vi "CalcHum.vi"(8 "error in (no error)":errorcluster, 10 "Adc_Hum":i32, 11 "BME68x in":refnum<class "BME680.lvclass">) -> (0 "error out":errorcluster, 2 "Hum":i32, 3 "BME68x out":refnum<class "BME680.lvclass">)   [LabVIEW 2022 SP3, in "BME680.lvlib" / "BME680.lvclass"]
uses:
  BME680.lvclass
  BME680.lvclass/BME680.ctl
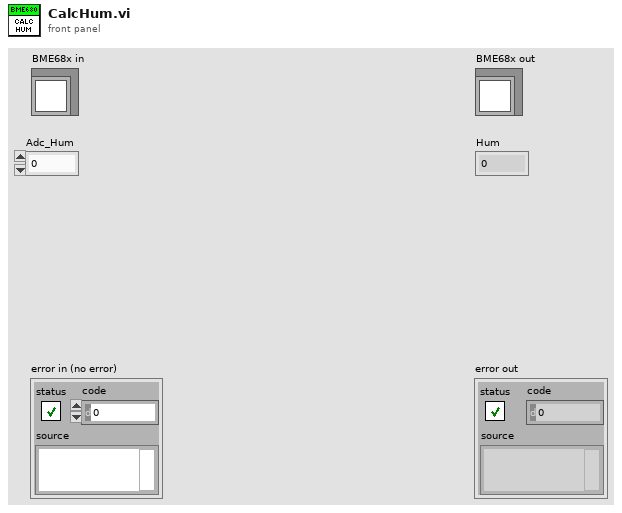
[diagram p1: front panel]
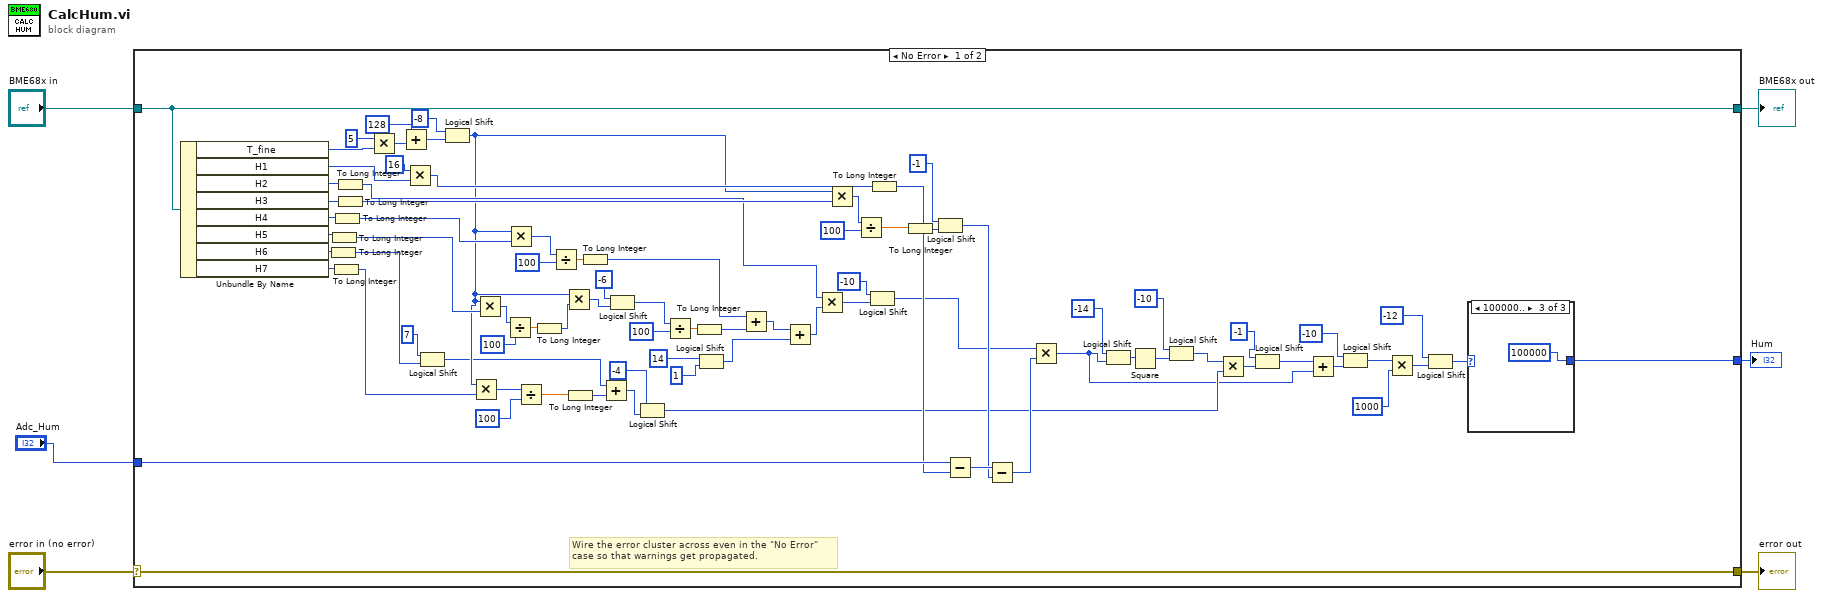
[diagram p0: block diagram]
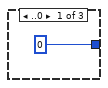
[diagram p2: hidden frame]
diagram:
  n1 = case shown="No Error" "error in (no error)" {
    selector: "error in (no error)" -> [w88 w93]
    tunnel: [w88 w93] -> w5
    tunnel: [w8 w92] -> w3
    tunnel: "BME68x in" -> [w8 w92]
    tunnel: "Adc_Hum" -> [w82 _]
    tunnel: [w7 _] -> w1
    frame No Error {
      # "Wire the error cluster across even in the \"No Error\"\ncase so that warnings get propagated."
      n2 = Unbundle By Name(w8) -> ("T_fine"=w87:i32, "H1"=w81:u16, "H2"=w52:u16, "H3"=w76:u8, "H4"=w66:u8, "H5"=w67:u8, "H6"=w48:u8, "H7"=w47:u8)
      n3 = To Long Integer(number=w48) -> (32bit integer=w32:i32)
      n4 = To Long Integer(number=w67) -> (32bit integer=w64:i32)
      n5 = To Long Integer(number=w47) -> (32bit integer=w45:i32)
      n6 = To Long Integer(number=w66) -> (32bit integer=w65:i32)
      n7 = To Long Integer(number=w52) -> (32bit integer=w51:i32)
      n8 = To Long Integer(number=w76) -> (32bit integer=w75:i32)
      n9 = Multiply(x=5, y=w87) -> (x*y=w85:i32)
      n10 = Add(x=128, y=w85) -> (x+y=w24:i32)
      n11 = Multiply(x=u16 16, y=w81) -> (x*y=w79:u16)
      n12 = Logical Shift(y=7 ("x"), x=w32) -> (x << y=w41:i32)
      n13 = Logical Shift(y=i16 -8, x=w24) -> (x << y=w46:i32)
      n14 = Multiply(x=w46, y=w45) -> (x*y=w42:i32)
      n15 = Multiply(x=w46, y=w64) -> (x*y=w61:i32)
      n16 = Divide(x=w61, y=100) -> (x/y=w62:dbl)
      n17 = Multiply(x=w46, y=w65) -> (x*y=w69:i32)
      n18 = Divide(x=w42, y=100) -> (x/y=w43:dbl)
      n19 = To Long Integer(number=w62) -> (32bit integer=w57:i32)
      n20 = Divide(x=w69, y=100) -> (x/y=w68:dbl)
      n21 = Multiply(x=w46, y=w57) -> (x*y=w26:i32)
      n22 = To Long Integer(number=w43) -> (32bit integer=w40:i32)
      n23 = To Long Integer(number=w68) -> (32bit integer=w33:i32)
      n24 = Add(x=w41, y=w40) -> (x+y=w30:i32)
      n25 = Logical Shift(y=-6 ("x"), x=w26) -> (x << y=w58:i32)
      n26 = Logical Shift(y=-4 ("x"), x=w30) -> (x << y=w37:i32)
      n27 = Divide(x=w58, y=100) -> (x/y=w59:dbl)
      n28 = To Long Integer(number=w59) -> (32bit integer=w56:i32)
      n29 = Logical Shift(y=14 ("x"), x=1 ("y")) -> (x << y=w55:i32)
      n30 = Add(x=w33, y=w56) -> (x+y=w54:i32)
      n31 = Add(x=w54, y=w55) -> (x+y=w53:i32)
      n32 = Multiply(x=w51, y=w53) -> (x*y=w23:i32)
      n33 = Multiply(x=w46, y=w75) -> (x*y=w73:i32)
      n34 = Divide(x=w73, y=100) -> (x/y=w72:dbl)
      n35 = Logical Shift(y=-10 ("x"), x=w23) -> (x << y=w49:i32)
      n36 = To Long Integer(number=w79) -> (32bit integer=w78:i32)
      n37 = To Long Integer(number=w72) -> (32bit integer=w21:i32)
      n38 = Logical Shift(y=-1 ("x"), x=w21) -> (x << y=w71:i32)
      n39 = Subtract(x=w82, y=w78) -> (x-y=w77:i32)
      n40 = Subtract(x=w77, y=w71) -> (x-y=w50:i32)
      n41 = Multiply(x=w49, y=w50) -> (x*y=w14:i32)
      n42 = Logical Shift(y=-14 ("x"), x=w14) -> (x << y=w39:i32)
      n43 = Square(x=w39) -> (x^2=w18:i32)
      n44 = Logical Shift(y=-10 ("x"), x=w18) -> (x << y=w38:i32)
      n45 = Multiply(x=w38, y=w37) -> (x*y=w16:i32)
      n46 = Logical Shift(y=-1 ("x"), x=w16) -> (x << y=w13:i32)
      n47 = Add(x=w13, y=w14) -> (x+y=w12:i32)
      n48 = Logical Shift(y=-10 ("x"), x=w12) -> (x << y=w36:i32)
      n49 = Multiply(x=w36, y=1000) -> (x*y=w10:i32)
      n50 = Logical Shift(y=-12 ("x"), x=w10) -> (x << y=w34:i32)
      n51 = case shown="100000.." w34 {
        selector: w34 -> [_ w90 _]
        tunnel: [0 w90 100000] -> w7
        frame ..0 {
        }
        frame 1..99999 {
        }
        frame 100000.. {
        }
      }
    }
    frame Error {
    }
  }
  "error out" <- w5
  "BME68x out" <- w3
  "Hum" <- w1
